vi "Write Default Dot Cluster.vi"(8 "error in (no error)":errorcluster, 10 "Default Dot":T1, 11 "Dot Settings in":refnum<class "Dot Settings.lvclass">) -> (0 "error out":errorcluster, 3 "Dot Settings out":refnum<class "Dot Settings.lvclass">)   [LabVIEW 2019, in "Dot Settings.lvclass"]
uses:
  Dot Settings.lvclass
  TypeDefs/Default Dot Cluster.ctl
  TypeDefs/Action.ctl
  Dot Settings.lvclass/Dot Settings.ctl
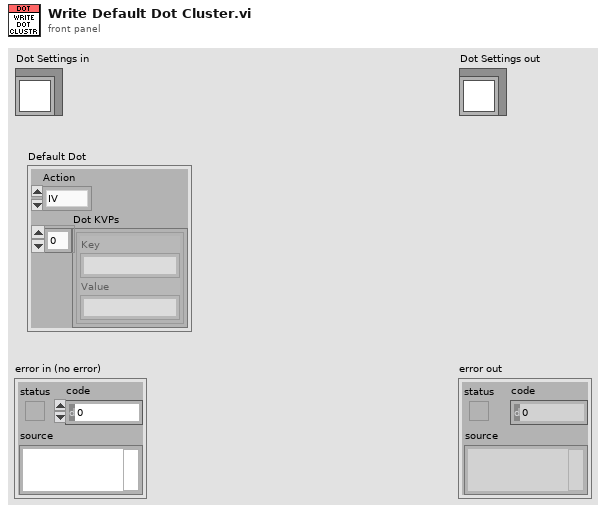
[diagram p1: front panel]
types:
  T1 = typedef "Dot Settings.lvclass/Default Dot Cluster.ctl" = cluster{"Action":T2, "Dot KVPs":cluster{"Key":string, "Value":string}[]}
  T2 = typedef "Dot Settings.lvclass/Action.ctl" = enum16{"IV", "QD"}
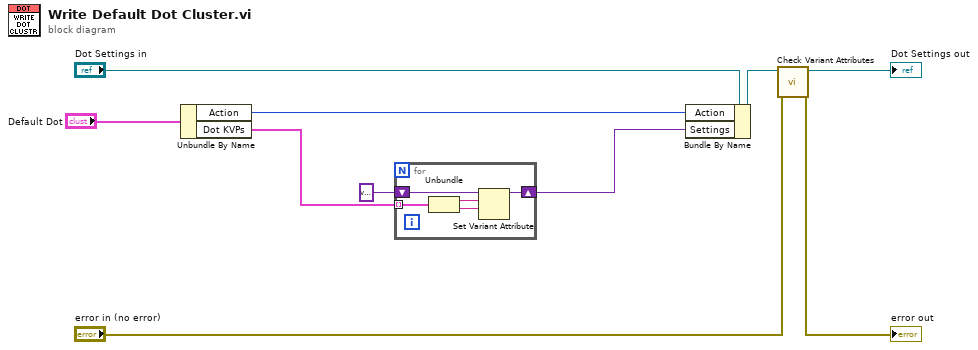
[diagram p0: block diagram]
diagram:
  n1 = Unbundle By Name("Default Dot") -> ("Action"=w8:T2, "Dot KVPs"=w6:cluster{"Key":string, "Value":string}[])
  n2 = for {
    shift-right: [w11] -> w5
    shift-left: variant -> [w15]
    tunnel: w6 -> [w14] mode=indexing
    n3 = Unbundle(w14) -> ("Key"=w13:string, "Value"=w12:string)
    n4 = Set Variant Attribute(Variant=w15, name=w13, value=w12) -> (Variant out=w11:variant)  [unwired: 1 in, 2 out]
  }
  n5 = Bundle By Name(cluster="Dot Settings in", "Action"=w8, "Settings"=w5) -> (w4:refnum<class "Dot Settings.lvclass">)
  n6 = call "Check Variant Attributes.vi"("error in (no error)"="error in (no error)", "Dot Settings in"=w4) -> ("error out"=→"error out":errorcluster, "Dot Settings out"=→"Dot Settings out":refnum<class "Dot Settings.lvclass">)  [unwired: 8 in]
